vi "Configure Measurement.vi"(6 "Manual Range (1.0)":dbl=1.0, 8 "error in (no error)":errorcluster, 9 "Auto Range (T:Enable)":bool=TRUE, 10 "Function (0: DC Volts)":u16(ring) items=["DC Volts", "AC Volts", "DC Current", "AC Current"], 11 "VISA resource name":refnum<visa-resource-name>) -> (0 "error out":errorcluster, 3 "VISA resource name out":refnum<visa-resource-name>)   [LabVIEW 2017, in "DmmPwr Simulator.lvlib"]
doc: "Configures the measurement type, and range on the instrument."
uses:
  DmmPwr Simulator.lvlib
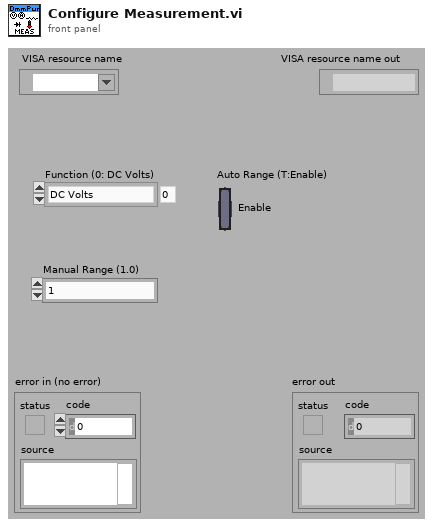
[diagram p1: front panel]
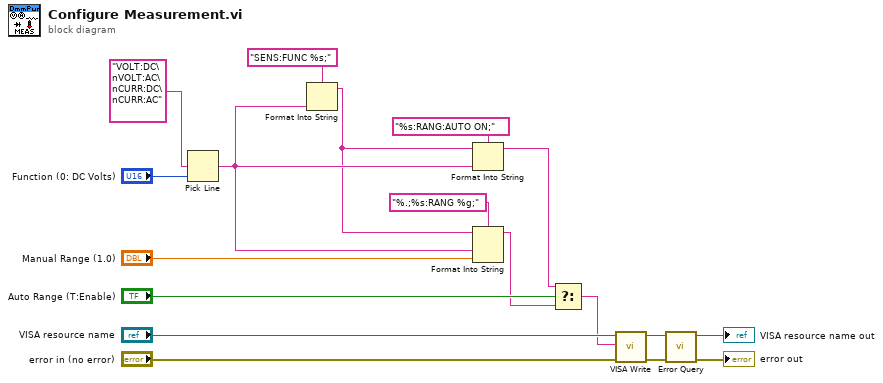
[diagram p0: block diagram]
diagram:
  n1 = Pick Line(multi-line string="VOLT:DC\nVOLT:AC\nCURR:DC\nCURR:AC" ("Function"), line index="Function (0: DC Volts)") -> (output string=w10:string)  [unwired: 1 in]
  n2 = Format Into String(format string="SENS:FUNC %s;" ("Select Function"), w10) -> (resulting string=w6:string)  [unwired: 2 in, 1 out]
  n3 = Format Into String(format string="%s:RANG:AUTO ON;" ("Auto Range"), initial string=w6, w10) -> (resulting string=w8:string)  [unwired: 1 in, 1 out]
  n4 = Format Into String(format string="%.;%s:RANG %g;" ("Manual Range"), initial string=w6, w10, "Manual Range (1.0)") -> (resulting string=w7:string)  [unwired: 1 in, 1 out]
  n5 = Select(t=w8, s="Auto Range (T:Enable)", f=w7) -> (s? t:f=w1:string)
  n6 = call "VISA Write.vi"("error in"="error in (no error)", "write buffer"=w1, "VISA resource name"="VISA resource name") -> ("error out"=w4:errorcluster, "VISA resource name out"=w3:refnum<visa-resource-name>)  [unwired: 6 in, 1 out]
  n7 = call "Error Query.vi"("error in (no error)"=w4, "VISA resource name"=w3) -> ("error out"=→"error out":errorcluster, "VISA resource name out"=→"VISA resource name out":refnum<visa-resource-name>)  [unwired: 6 in, 2 out]
